vi "Shuffle Test Methods.vi"(10 "VI refs in":refnum<vi>[](array[refnum]), 11 "Slave Test Runner in":refnum<class "Slave Test Runner.lvclass">) -> (2 "shuffled array":refnum<vi>[](array[refnum]), 3 "Slave Test Runner out":refnum<class "Slave Test Runner.lvclass">)   [LabVIEW 2020, in "Slave Test Runner.lvclass"]
uses:
  Slave Test Runner.lvclass
  Slave Test Runner.lvclass/Slave Test Runner.ctl
  2fc74b80-6deb-4f17-a78e-34401938511c.vi
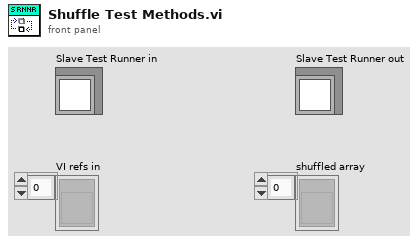
[diagram p1: front panel]
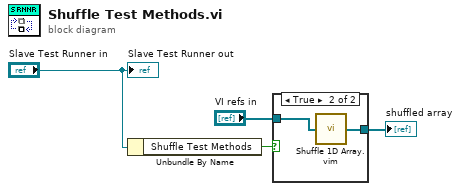
[diagram p0: block diagram]
diagram:
  n1 = Unbundle By Name("Slave Test Runner in") -> ("Shuffle Test Methods"=w4:bool)
  n2 = case shown="True" w4 {
    tunnel: "VI refs in" -> [w5 w7]
    tunnel: [w5 w6] -> w3
    frame False {
    }
    frame True {
      n3 = call "Shuffle 1D Array.vim"("array"=w7) -> ("shuffled array"=w6:refnum<vi>[])  [unwired: 4 in]
    }
  }
  "shuffled array" <- w3
  "Slave Test Runner out" <- "Slave Test Runner in"
